vi "Grabber Control.vi"(11 "Grabber Sensor In":bool) -> (3 "PWM 8+9 Output":dbl)   [LabVIEW 2011]
uses:
  Robot Global Data.vi
panel:
  in  "Gripper Wait":u32=250
  out "Delay Run":bool
  in  "Gripper State":dbl
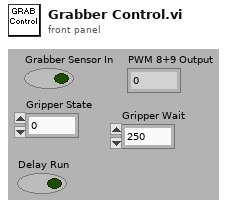
[diagram p1: front panel]
types:
  T1 = cluster{"Axis 1":dbl, "Axis 2":dbl, "Axis 3":dbl, "Axis 4":dbl, "Axis 5":dbl, "Axis 6":dbl, "Button 1":bool, "Button 2":bool, "Button 3":bool, "Button 4":bool, "Button 5":bool, "Button 6":bool, "Button 7":bool, "Button 8":bool, "Button 9":bool, "Button 10":bool, "Button 11":bool, "Button 12":bool}
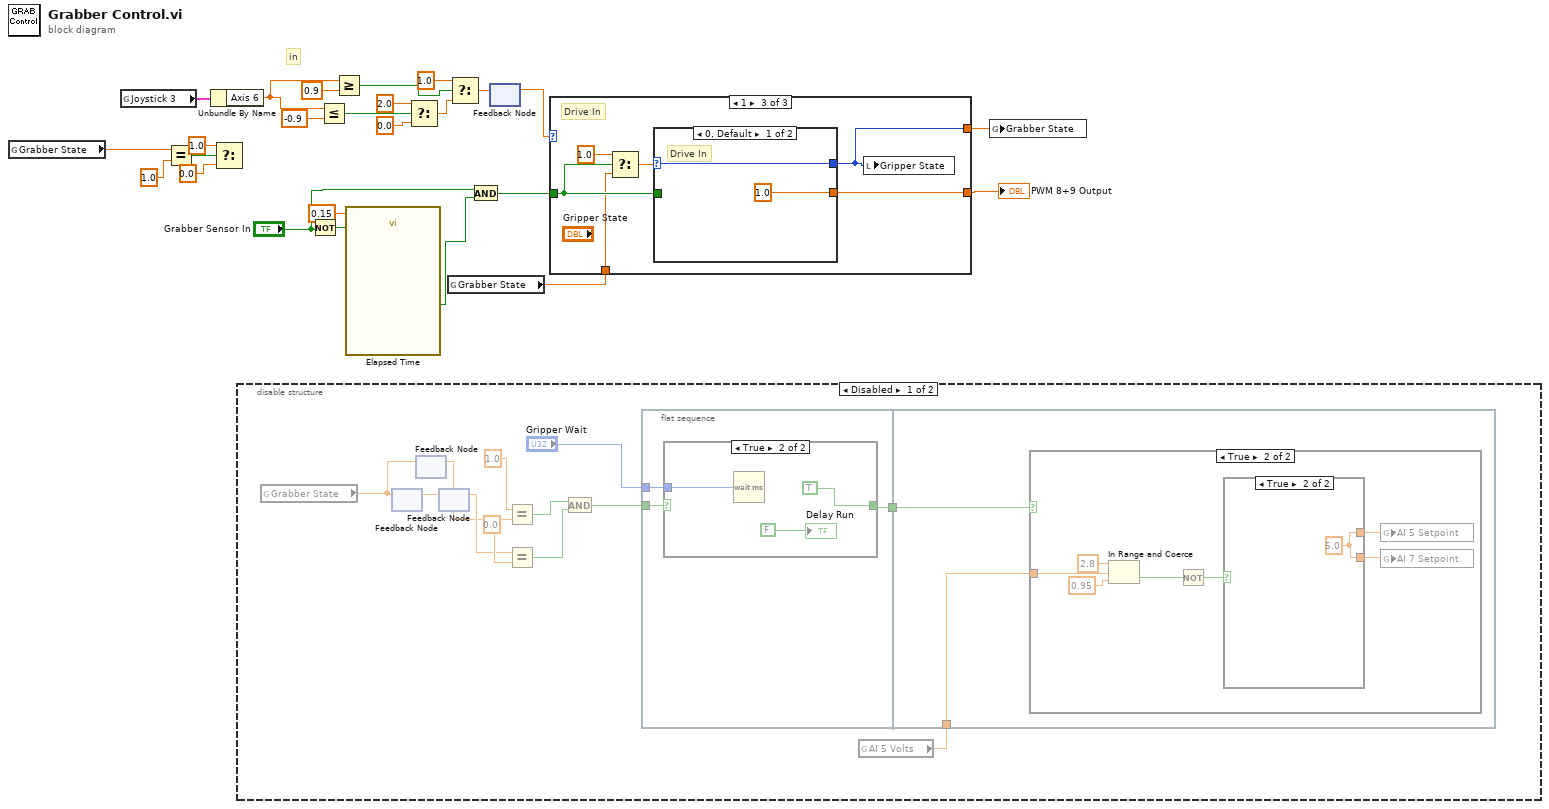
[diagram p0: block diagram]
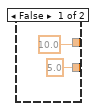
[diagram p4: hidden frame]
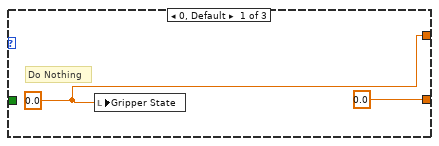
[diagram p6: hidden frame]
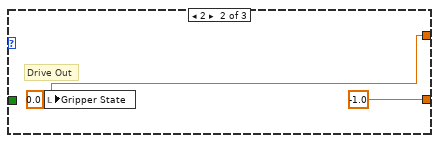
[diagram p7: hidden frame]
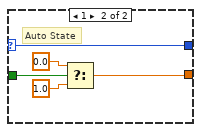
[diagram p8: hidden frame]
diagram:
  # "in"
  n1 = global read "Robot Global Data.vi" "Grabber State"() -> (w9:dbl)
  n2 = global read "Robot Global Data.vi" "Joystick 3"() -> (w25:T1)
  n3 = Equal?(x=w9, y=1.0) -> (x = y?=w18:bool)
  n4 = Unbundle By Name(w25) -> ("Axis 6"=w12:dbl)
  n5 = Select(t=1.0, s=w18, f=0.0) -> ()  [unwired: 1 out]
  n6 = disable-structure shown="Disabled" {
    frame Disabled {
      n7 = global read "Robot Global Data.vi" "Grabber State"() -> (w27:dbl)
      n8 = feedback-in #1(w27) -> ()
      n9 = feedback #1() -> (w30:dbl)  [unwired: 1 out]
      n10 = feedback-in #2(w27) -> ()
      n11 = feedback #2() -> (w28:dbl)  [unwired: 1 out]
      n12 = feedback-in #3(w30) -> ()
      n13 = feedback #3() -> (w29:dbl)  [unwired: 1 out]
      n14 = Equal?(x=1.0, y=w28) -> (x = y?=w34:bool)
      n15 = Equal?(x=w29, y=0.0) -> (x = y?=w33:bool)
      n16 = And(x=w34, y=w33) -> (x .and. y?=w32:bool)
      n17 = flat-sequence {
        tunnel: w32 -> [w40]
        tunnel: "Gripper Wait" -> [w39]
        tunnel: [w38] -> w37
        tunnel: w37 -> [w46]
        tunnel: w26 -> [w45]
        frame #0 {
          n18 = case shown="True" w40 {
            selector: w40 -> [w41 _]
            tunnel: w39 -> [_ w43]
            tunnel: [w41 TRUE ("Delay Run")] -> w38
            frame False {
              # "nothing"
            }
            frame True {
              n19 = Wait (ms)(milliseconds to wait=w43) -> ()  [unwired: 1 out]
              "Delay Run" <- FALSE ("Delay Run")
            }
          }
        }
        frame #1 {
          n20 = case shown="True" w46 {
            tunnel: w45 -> [_ w51]
            frame False {
            }
            frame True {
              n21 = In Range and Coerce(upper limit=2.8, x=w51, lower limit=0.95 ("y")) -> (In Range?=w49:bool)  [unwired: 1 out]
              n22 = Not(x=w49) -> (.not. x?=w50:bool)
              n23 = case shown="True" w50 {
                tunnel: [10.0 ("AI 5 Setpoint") w56] -> w48
                tunnel: [5.0 ("AI 7 Setpoint") w56] -> w47
                frame False {
                }
                frame True {
                  w56 = 5.0 ("AI 7 Setpoint")
                }
              }
              n24 = global write "Robot Global Data.vi" "AI 5 Setpoint"(w48) -> ()
              n25 = global write "Robot Global Data.vi" "AI 7 Setpoint"(w47) -> ()
            }
          }
        }
      }
      n26 = global read "Robot Global Data.vi" "AI 5 Volts"() -> (w26:dbl)
    }
    frame Enabled {
    }
  }
  n27 = Not(x="Grabber Sensor In") -> (.not. x?=w4:bool)
  n28 = Less Or Equal?(x=w12, y=-0.9) -> (x <= y?=w13:bool)
  n29 = Greater Or Equal?(x=w12, y=0.9) -> (x >= y?=w14:bool)
  n30 = call "Elapsed Time"("Time Target (s)"=0.15, "Reset"=w4) -> ("Time has Elapsed"=w6:bool)  [unwired: 3 in, 14 out]
  n31 = Select(t=2.0, s=w13, f=0.0) -> (s? t:f=w22:dbl)
  n32 = global read "Robot Global Data.vi" "Grabber State"() -> (w1:dbl)
  n33 = Select(t=1.0, s=w14, f=w22) -> (s? t:f=w24:dbl)
  n34 = And(x="Grabber Sensor In", y=w6) -> (x .and. y?=w8:bool)
  n35 = feedback-in #4(w24) -> ()
  n36 = feedback #4() -> (w16:dbl)  [unwired: 1 out]
  n37 = case shown="1" w16 {
    tunnel: w8 -> [_ _ w66]
    tunnel: [0.0 ("f") -1.0 ("f") w63] -> w20
    tunnel: [w57 w59 w62] -> w3
    tunnel: w1 -> [_ _ w61]
    frame 0, Default {
      w57 = 0.0 ("Gripper State")
      # "Do Nothing"
      n38 = local write "Gripper State"(w57) -> ()
    }
    frame 2 {
      w59 = 0.0 ("Gripper State")
      # "Drive Out"
      n39 = local write "Gripper State"(w59) -> ()
    }
    frame 1 {
      # "Drive In"
      n40 = Select(t=1.0, s=w66, f=w61) -> (s? t:f=w64:dbl)
      n41 = case shown="0, Default" w64 {
        selector: w64 -> [w68 w70]
        tunnel: w66 -> [_ w73]
        tunnel: [w68 w70] -> w62
        tunnel: [1.0 ("f") w69] -> w63
        frame 0, Default {
          # "Drive In"
        }
        frame 1 {
          # "Auto State"
          n42 = Select(t=0.0, s=w73, f=1.0) -> (s? t:f=w69:dbl)
        }
      }
      n43 = local write "Gripper State"(w62) -> ()
    }
  }
  "PWM 8+9 Output" <- w20
  n44 = global write "Robot Global Data.vi" "Grabber State"(w3) -> ()
